vi "VerifyCommandNumber.vi"(8 "error in":errorcluster, 10 "Command #(From Response)":u32, 11 "Command #":u8) -> (0 "error out":errorcluster)   [LabVIEW 2020, in "driver_flodx_pressure.lvlib"]
uses:
  <instrlib>/RxnRover/FloDx Pressure Driver/driver_flodx_pressure.lvlib
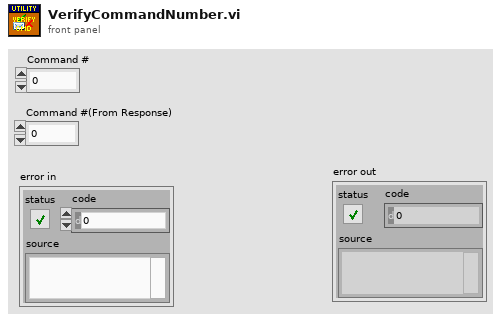
[diagram p1: front panel]
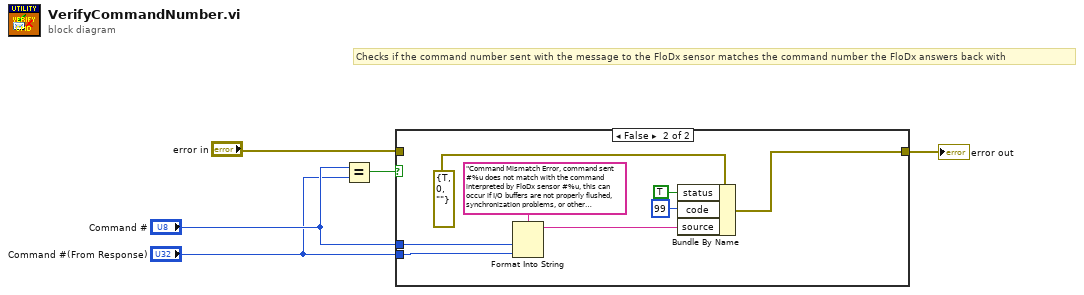
[diagram p0: block diagram]
diagram:
  # "Checks if the command number sent with the message to the FloDx sensor matches the command number the FloDx answers back with"
  n1 = Equal?(x="Command #", y="Command #(From Response)") -> (x = y?=w4:bool)
  n2 = case shown="False" w4 {
    tunnel: [w6 w13] -> w2
    tunnel: "error in" -> [w6 _]
    tunnel: "Command #" -> [_ w8]
    tunnel: "Command #(From Response)" -> [_ w7]
    frame True {
    }
    frame False {
      n3 = Format Into String(format string="Command Mismatch Error, command sent #%u does not match with the command interpreted by FloDx sensor #%u, this can occur if I/O buffers are not properly flushed, synchronization problems, or other communication issues", w8, w7) -> (resulting string=w9:string)  [unwired: 2 in, 1 out]
      n4 = Bundle By Name(cluster=errorcluster {"status"=TRUE, "code"=0, "source"=""} ("error IO"), "status"=TRUE, "code"=99, "source"=w9) -> (w13:errorcluster)
    }
  }
  "error out" <- w2
